vi "Gauss_Fit.vi"(0 "Freq_Data":dbl[](array[numeric]), 1 "Scptrm_Data":dbl[](array[numeric]), 2 "Freqs":T1={"Ffitlo / MHz"=70.0, "Fcentre / MHz"=80.0, "Ffithi / MHz"=90.0, "LLest / MHz"=2.6187499999999915, "Peak Est / nW"=0.0, "Gau stdev / MHz "=2.6187499999999915}) -> (3 "freq_fit_data":dbl[](array[numeric]), 4 "spctrm_fit_data":dbl[](array[numeric]), 5 "a_pars":dbl[](array[numeric])=[0.7072584069399376, 80.0, 1.7560129064005117], 6 "gof_stats":dbl[](array[numeric])=[3199.0, 1.0009386733416772, 0.954874518705434, 0.4817149539059473])   [LabVIEW 2020]
doc: "Fit a Lorentzian to measured LLM spectral data\n\nFreq_Data assumed in units of MHz\nSpctrm_Data assumed in units of dBm\nFfitlo, Ffithi in units of MHz must be inside range of Freq_Data\nFit_Data output in units of dBm\na_pars = [Amplitude, Centre Frequency [MHz], Linewidth [MHz] ]\ngof_stats = [chi^{2}, chi^{2} / nu, R^{2}, gof probability]\n\nR. Sheehan 9 - 11 - 2021"
uses:
  C++/Fitting/Non_Lin_Fit/Release/Non_Lin_Fit.dll
panel:
  # "Amp. Par\n\nAOM Freq / MHz\n\nStd. Dev. / MHz"
  # "chi^{2} for the fit\n\nchi^{2} / nu\n\nR^{2}\n\nGOF"
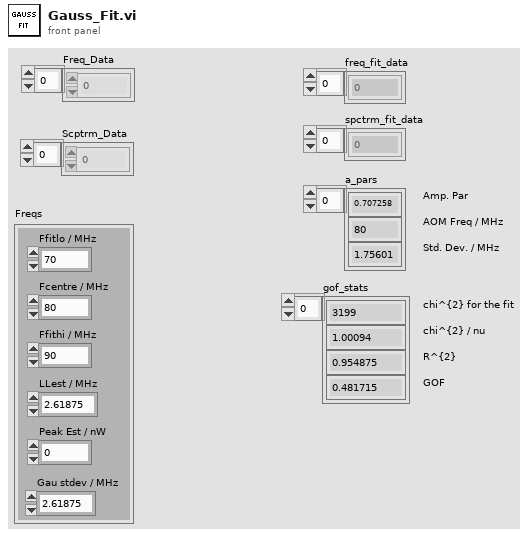
[diagram p1: front panel]
types:
  T1 = cluster{"Ffitlo / MHz":dbl, "Fcentre / MHz":dbl, "Ffithi / MHz":dbl, "LLest / MHz":dbl, "Peak Est / nW":dbl, "Gau stdev / MHz ":dbl}
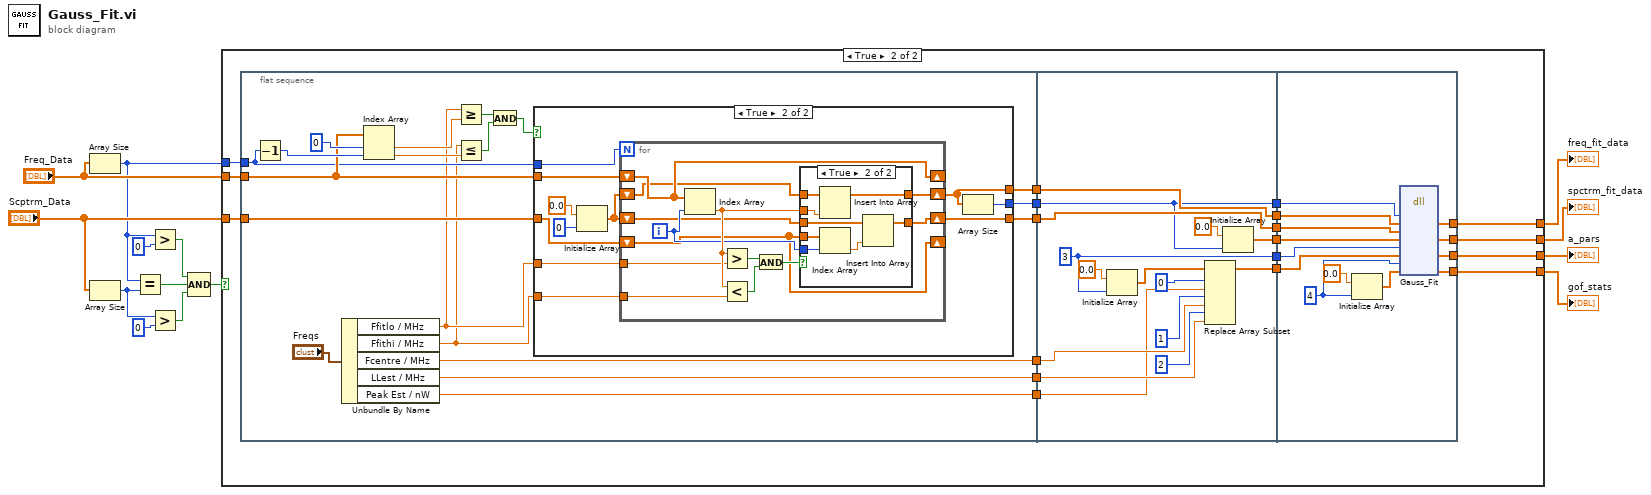
[diagram p0: block diagram]
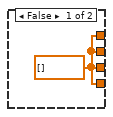
[diagram p2: hidden frame]
diagram:
  n1 = Array Size(array="Freq_Data") -> (size(s)=w9:i32)
  n2 = Array Size(array="Scptrm_Data") -> (size(s)=w10:i32)
  n3 = Equal?(x=w9, y=w10) -> (x = y?=w7:bool)
  n4 = Greater?(x=w9, y=0) -> (0:w8:bool)
  n5 = Greater?(x=w10, y=0) -> (0:w6:bool)
  n6 = Compound Arithmetic op=AND(w8, w7, w6) -> (w5:bool)
  n7 = case shown="True" w5 {
    tunnel: "Freq_Data" -> [_ w34]
    tunnel: "Scptrm_Data" -> [_ w33]
    tunnel: w9 -> [_ w32]
    tunnel: [w15 w20] -> w4
    tunnel: [w15 w19] -> w3
    tunnel: [w15 w18] -> w2
    tunnel: [w15 w17] -> w1
    frame False {
      w15 = dbl[] [] ("freq_data")
    }
    frame True {
      n8 = flat-sequence {
        tunnel: w34 -> [w46]
        tunnel: w33 -> [w45]
        tunnel: w32 -> [w44]
        tunnel: [w43] -> w31
        tunnel: [w42] -> w29
        tunnel: [w41] -> w27
        tunnel: [w37] -> w22
        tunnel: [w36] -> w21
        tunnel: [w35] -> w16
        tunnel: w31 -> [w94]
        tunnel: [w99] -> w30
        tunnel: w29 -> [w99]
        tunnel: [w98] -> w28
        tunnel: w27 -> [w98]
        tunnel: [w97] -> w26
        tunnel: [w96] -> w25
        tunnel: [w95] -> w24
        tunnel: [w94] -> w23
        tunnel: w22 -> [w93]
        tunnel: w21 -> [w92]
        tunnel: w16 -> [w91]
        tunnel: w30 -> [w115]
        tunnel: w28 -> [w114]
        tunnel: w26 -> [w113]
        tunnel: w25 -> [w112]
        tunnel: w24 -> [w111]
        tunnel: w23 -> [w110]
        tunnel: [w109] -> w20
        tunnel: [w108] -> w19
        tunnel: [w107] -> w18
        tunnel: [w106] -> w17
        frame #0 {
          n9 = Decrement(x=w44) -> (x-1=w51:i32)
          n10 = Unbundle By Name("Freqs") -> ("Ffitlo / MHz"=w39:dbl, "Ffithi / MHz"=w38:dbl, "Fcentre / MHz"=w37:dbl, "LLest / MHz"=w36:dbl, "Peak Est / nW"=w35:dbl)
          n11 = Index Array(array=w46, index #1=0 ("index"), index #2=w51) -> (element #1=w52:dbl, element #2=w50:dbl)
          n12 = Greater Or Equal?(x=w39, y=w52) -> (x >= y?=w49:bool)
          n13 = Less Or Equal?(x=w38, y=w50) -> (x <= y?=w48:bool)
          n14 = And(x=w49, y=w48) -> (x .and. y?=w47:bool)
          n15 = case shown="True" w47 {
            tunnel: w45 -> [w54 w67]
            tunnel: [w55 w63] -> w42
            tunnel: [w54 w62] -> w41
            tunnel: [w56 w61] -> w43
            tunnel: w39 -> [_ w60]
            tunnel: w46 -> [w55 w59]
            tunnel: w38 -> [_ w58]
            tunnel: w44 -> [w56 w57]
            frame False {
            }
            frame True {
              n16 = Initialize Array(0.0 ("element"), 0 ("dimension size")) -> (w64:dbl[])
              n17 = for {
                N: w57 -> [_]
                shift-right: [w80] -> _
                shift-left: w59 -> [w80]
                shift-right: [w74] -> _
                shift-left: w67 -> [w74]
                shift-right: [w72] -> w63
                shift-left: w64 -> [w73]
                shift-right: [w70] -> w62
                shift-left: w64 -> [w71]
                tunnel: w60 -> [w69]
                tunnel: w58 -> [w68]
                i -> [w75]
                n18 = Index Array(array=w80, index=w75) -> (element=w76:dbl)
                n19 = Greater?(x=w76, y=w69) -> (0:w79:bool)
                n20 = Less?(x=w76, y=w68) -> (x < y?=w78:bool)
                n21 = And(x=w79, y=w78) -> (x .and. y?=w77:bool)
                n22 = case shown="True" w77 {
                  tunnel: w76 -> [_ w86]
                  tunnel: w75 -> [_ w90]
                  tunnel: w74 -> [_ w89]
                  tunnel: w73 -> [w82 w88]
                  tunnel: [w82 w87] -> w72
                  tunnel: w71 -> [w81 w85]
                  tunnel: [w81 w84] -> w70
                  frame False {
                  }
                  frame True {
                    n23 = Insert Into Array(array=w88, new element=w86) -> (w87:dbl[])  [unwired: 1 in]
                    n24 = Index Array(array=w89, index=w90) -> (element=w83:dbl)
                    n25 = Insert Into Array(array=w85, new element=w83) -> (w84:dbl[])  [unwired: 1 in]
                  }
                }
              }
              n26 = Array Size(array=w63) -> (size(s)=w61:i32)
            }
          }
        }
        frame #1 {
          w95 = 3 ("Npars")
          n27 = Initialize Array(0.0 ("element"), w95) -> (w105:dbl[])
          n28 = Replace Array Subset(array=w105, new element #1=w91, index #1=0 ("index"), new element #2=w93, index #2=1 ("index"), new element #3=w92, index #3=2 ("index")) -> (w96:dbl[])
          n29 = Initialize Array(0.0 ("element"), w94) -> (w97:dbl[])
        }
        frame #2 {
          w118 = 4 ("Nstats")
          n30 = Initialize Array(0.0 ("element"), w118) -> (w117:dbl[])
          n31 = dll-call lib="C:/Users/robertsheehan/Programming/C++/Fitting/Non_Lin_Fit/Release/Non_Lin_Fit.dll" fn="Gauss_Fit"("n_data"=w110, "freq_data"=w115, "spctrm_data"=w114, "fit_data"=w113, "n_pars"=w111, "a_pars"=w112, "n_stats"=w118, "gof_stats"=w117) -> ("freq_data"=w109:dbl[], "fit_data"=w108:dbl[], "a_pars"=w107:dbl[], "gof_stats"=w106:dbl[])  [unwired: 8 in, 2 out]
        }
      }
    }
  }
  "freq_fit_data" <- w4
  "spctrm_fit_data" <- w3
  "a_pars" <- w2
  "gof_stats" <- w1
